vi "Test Set Row Values DateTime.vi"(11 "Test Case In":refnum<class "Test Open Xml.lvclass">) -> (0 "error out":errorcluster, 3 "Test Case Out":refnum<class "Test Open Xml.lvclass">)   [LabVIEW 2025, in "Test Open Xml.lvclass"]
uses:
  Test Open Xml.lvclass
  C:/Program Files/National Instruments/LabVIEW 2025/vi.lib/Astemes/LUnit/Test Case.lvclass
  Source/Cell DataType.ctl
  <vilib>/Astemes/LUnit/Test Case.lvclass/Test Case.ctl
  6bd0ddee-c4a9-43dd-9f12-e32be91059bb.vi
  efeba741-6930-4178-aa8a-aa8c96a7f46d.vi
  <vilib>/Astemes/LUnit/Append Fail Result.vi
  <vilib>/Astemes/LUnit/Append Pass Result.vi
  <vilib>/Astemes/LUnit/Run In UI.vi
  <vilib>/Utility/error.llb/Clear Errors.vi
  <vilib>/Astemes/LUnit/Test Case.lvclass
  Source/Open Xml.lvlib
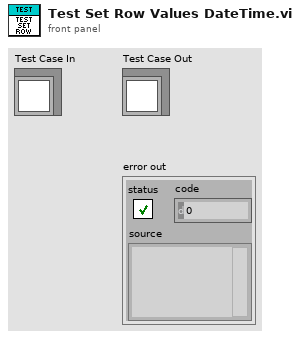
[diagram p1: front panel]
types:
  T1 = typedef "Open Xml.lvlib/Cell DataType.ctl" = enum16{"Void", "Boolean", "Number", "Error", "SharedString", "String", "InlineString", "Date"}
  T2 = cluster{"Number":dbl, "String":string, "Boolean":bool, "Time Stamp":timestamp, "Error":errorcluster}[]
  T3 = cluster{"Number":dbl, "String":string, "Boolean":bool, "Time Stamp":timestamp, "Error":errorcluster}
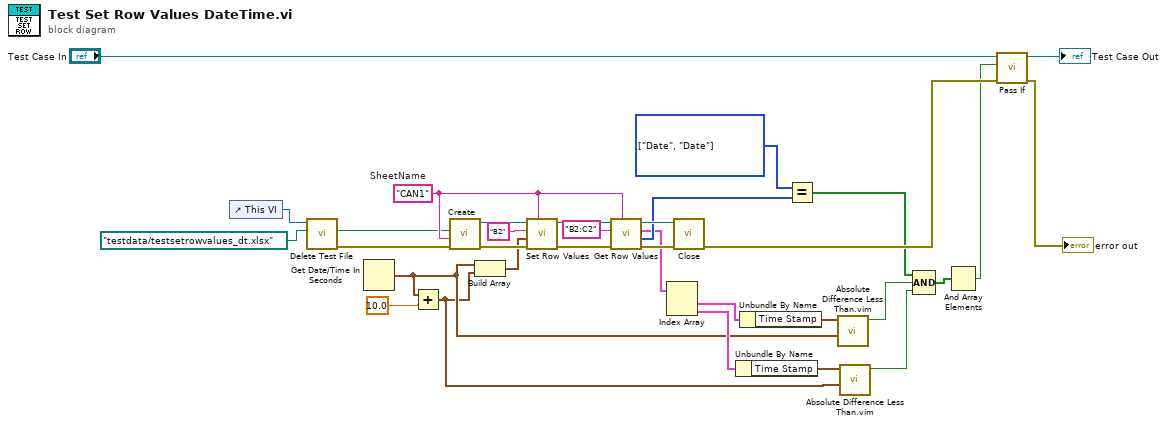
[diagram p0: block diagram]
diagram:
  w16 = T1[] [enum."Date", enum."Date"] items=["Void", "Boolean", "Number", "Error", "SharedString", "String", "InlineString", "Date"] ("x")
  w25 = "CAN1"  # SheetName
  n1 = control-ref of="This VI"() -> (w4:refnum<vi>)
  n2 = call "Delete Test File.vi"("name or relative path"=path "testdata/testsetrowvalues_dt.xlsx", "VI in"=w4) -> ("error out"=w1:errorcluster, "deleted path"=w2:path)  [unwired: 8 in]
  n3 = Get Date/Time In Seconds() -> (seconds since 1Jan1904=w9:timestamp)
  n4 = Add(x=w9, y=10.0) -> (x+y=w7:timestamp)
  n5 = call "Create.vi"("error in"=w1, "SheetName"=w25, "Path"=w2) -> ("error out"=w29:errorcluster, "SpreadsheetDoc"=w30:refnum<k24>)  [unwired: 7 in]
  n6 = Build Array(w9, w7) -> (w12:timestamp[])
  n7 = call "Set Row Values.vi"("Sheet Name"=w25, "error in"=w29, "Values"=w12, "Cell Address"="B2", "SpreadsheetDoc"=w30) -> ("error out"=w23:errorcluster, "SpreadsheetDoc out"=w22:refnum<k24>)  [unwired: 5 in]
  n8 = call "Get Row Values.vi"("Sheet Name"=w25, "error in"=w23, "Cell Addresses"="B2:C2" ("Cell Address"), "SpreadsheetDoc in"=w22) -> ("error out"=w27:errorcluster, "Types"=w21:T1[], "Cell Values"=w17:T2, "SpreadsheetDoc out"=w26:refnum<k24>)  [unwired: 4 in]
  n9 = Index Array(array=w17) -> (element #1=w15:T3, element #2=w14:T3)  [unwired: 2 in]
  n10 = call "Close.vi"("error in"=w27, "SpreadsheetDoc"=w26) -> ("error out"=w28:errorcluster)  [unwired: 9 in]
  n11 = Unbundle By Name(w14) -> ("Time Stamp"=w5:timestamp)
  n12 = Unbundle By Name(w15) -> ("Time Stamp"=w6:timestamp)
  n13 = Equal?(x=w16, y=w21) -> (x = y?=w20:bool[])
  n14 = call "Absolute Difference Less Than.vim"("Number 2"=w9, "Number 1"=w6) -> ("In Limit"=w11:bool)  [unwired: 9 in]
  n15 = call "Absolute Difference Less Than.vim"("Number 2"=w7, "Number 1"=w5) -> ("In Limit"=w10:bool)  [unwired: 9 in]
  n16 = Compound Arithmetic op=AND(w20, w11, w10) -> (w13:bool[])
  n17 = And Array Elements(Boolean array=w13) -> (logical AND=w24:bool)
  n18 = call <vilib>:"Pass If.vi"("error in (no error)"=w28, "Pass?"=w24, "LUnit Test Case In"="Test Case In") -> ("error out"=→"error out":errorcluster, "LUnit Test Case Out"=→"Test Case Out":refnum<class "Test Open Xml.lvclass">)  [unwired: 7 in]
